vi "Read MAP data file.vi"(11 "Data folder":path) -> (2 "File name":string, 3 "Map data ref":refnum<data-value>, 4 "Error Out":errorcluster)   [LabVIEW 2022 SP3]
uses:
  Datatypes/Map graph data.ctl
  <vilib>/Utility/error.llb/Error Cluster From Error Code.vi
  <vilib>/ErrorRing/Error Ring.xnode
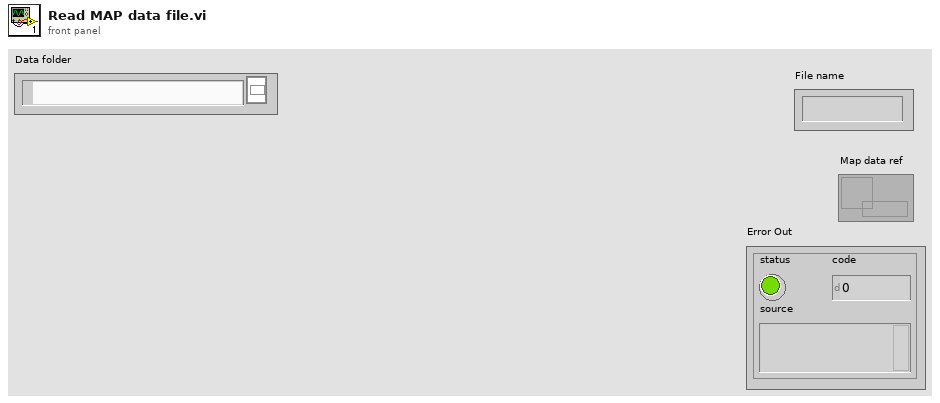
[diagram p1: front panel]
types:
  T1 = typedef "Map graph data.ctl" = cluster{"Field [T]":dbl[], "Intensity":dbl[][], "Start F [GHz]":dbl, "End F[GHz]":dbl, "BStart[T]":dbl, "Bend[T]":dbl, "Bsize":i32}
  T2 = enum16{"open", "open or create", "create or replace", "create", "open (read-only)"}
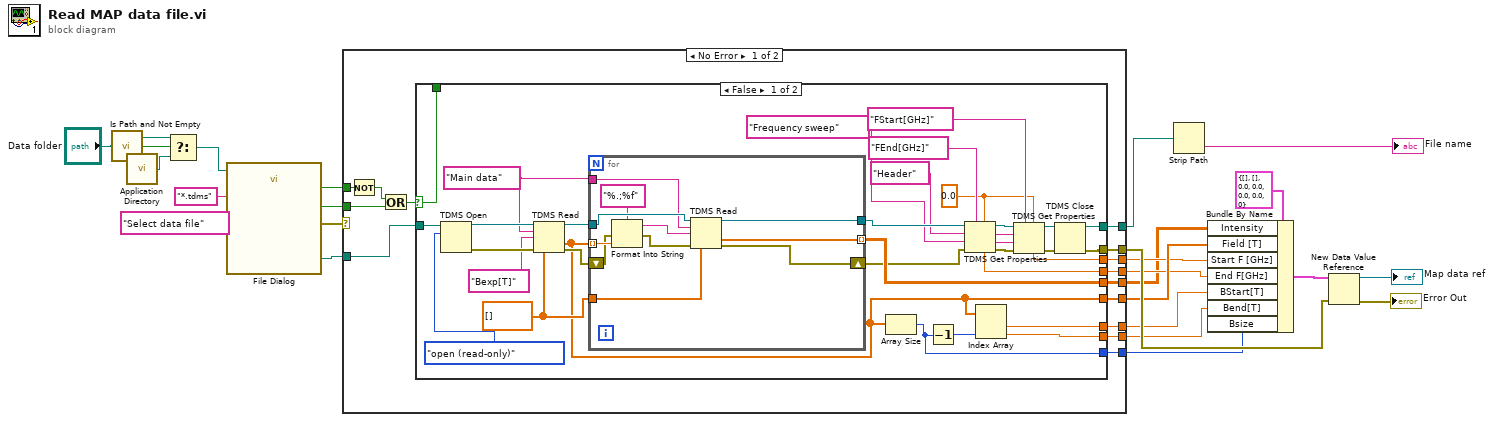
[diagram p0: block diagram]
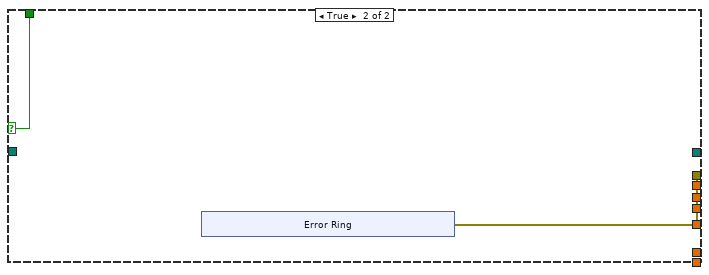
[diagram p2: hidden frame]
diagram:
  n1 = call <vilib>:"Is Path and Not Empty.vi"("path"="Data folder") -> ("Is Path and Not Empty?"=w18:bool)  [unwired: 4 in]
  n2 = call <vilib>:"Application Directory.vi"() -> ("Application Directory"=w15:path)
  n3 = Select(t="Data folder", s=w18, f=w15) -> (s? t:f=w16:path)
  n4 = call "File Dialog"("start path"=w16, "prompt"="Select data file", "pattern (all files)"="*.tdms") -> ("selected path"=w23:path, "exists"=w22:bool, "cancelled"=w21:bool, "error out"=w20:errorcluster)  [unwired: 9 in]
  n5 = case shown="No Error" w20 {
    selector: w20 -> [_ w89]
    tunnel: w23 -> [w38 _]
    tunnel: w22 -> [w37 _]
    tunnel: w21 -> [w34 _]
    tunnel: [w33 w89] -> w13
    tunnel: [w32 _] -> w11
    tunnel: [w31 _] -> w7
    tunnel: [w30 _] -> w9
    tunnel: [w29 _] -> w8
    tunnel: [w28 _] -> w6
    tunnel: [w27 _] -> w5
    tunnel: [w26 _] -> w4
    tunnel: [w25 _] -> w2
    frame No Error {
      n6 = Not(x=w37) -> (.not. x?=w36:bool)
      n7 = Or(x=w36, y=w34) -> (x .or. y?=w35:bool)
      n8 = case shown="False" w35 {
        selector: w35 -> [w71 w84]
        tunnel: w38 -> [w70 _]
        tunnel: [w71 w84] -> _
        tunnel: [w61 w83] -> w33
        tunnel: [w44 _] -> w32
        tunnel: [w60 _] -> w31
        tunnel: [w57 _] -> w29
        tunnel: [w46 _] -> w30
        tunnel: [w42 _] -> w28
        tunnel: [w41 _] -> w27
        tunnel: [w40 _] -> w26
        tunnel: [w39 _] -> w25
        frame False {
          w45 = "Main data"
          w47 = 0.0 ("Start F [GHz]")
          w64 = dbl[] []
          n9 = TDMS Open(10:T2."open (read-only)" ("operation (0:open)"), 11:w70) -> (0:w67:errorcluster, 3:w68:refnum<k34>)  [unwired: 5 in]
          n10 = TDMS Read(0:w68, 5:w45, 7:"Bexp[T]" ("channel name(s) in"), 11:w67, 12:w64) -> (4:w65:refnum<k34>, 10:w44:dbl[], 15:w63:errorcluster)  [unwired: 3 in, 3 out]
          n11 = for {
            tunnel: w65 -> [w79]
            tunnel: w44 -> [w82] mode=indexing
            tunnel: w64 -> [w74]
            tunnel: [w78] -> w60 mode=indexing
            tunnel: [w76] -> w62
            shift-right: [w77] -> w58
            shift-left: w63 -> [w75]
            tunnel: w45 -> [w73]
            n12 = Format Into String(format string="%.;%f", error in=w75, w82) -> (resulting string=w80:string, error out=w81:errorcluster)  [unwired: 1 in]
            n13 = TDMS Read(0:w79, 5:w73, 7:w80, 11:w81, 12:w74) -> (4:w76:refnum<k34>, 10:w78:dbl[], 15:w77:errorcluster)  [unwired: 3 in, 3 out]
          }
          n14 = Array Size(array=w44) -> (size(s)=w40:i32)
          n15 = Decrement(x=w40) -> (x-1=w43:i32)
          n16 = TDMS Get Properties(5:w47, 7:"FEnd[GHz]", 8:w58, 9:"Frequency sweep", 10:"Header" ("group name in"), 11:w62) -> (0:w52:errorcluster, 1:w48:string, 2:w49:string, 3:w59:refnum<k34>, 4:w57:dbl)  [unwired: 1 out]
          n17 = Index Array(array=w44, index #2=w43) -> (element #1=w42:dbl, element #2=w41:dbl)  [unwired: 1 in]
          n18 = TDMS Get Properties(5:w47, 7:"FStart[GHz]", 8:w52, 9:w48, 10:w49, 11:w59) -> (0:w53:errorcluster, 3:w54:refnum<k34>, 4:w46:dbl)  [unwired: 3 out]
          n19 = TDMS Close(8:w53, 11:w54) -> (0:w61:errorcluster, 3:w39:path)
        }
        frame True {
          n20 = xnode "Error Ring"() -> ("error out"=w83:errorcluster)
        }
      }
    }
    frame Error {
    }
  }
  n21 = Strip Path(path=w2) -> (name=→"File name":string)  [unwired: 1 out]
  n22 = Bundle By Name(cluster=T1 {"Field [T]"=[], "Intensity"=[], "Start F [GHz]"=0.0, "End F[GHz]"=0.0, "BStart[T]"=0.0, "Bend[T]"=0.0, "Bsize"=0} ("Cluster 2"), "Intensity"=w7, "Field [T]"=w11, "Start F [GHz]"=w9, "End F[GHz]"=w8, "BStart[T]"=w6, "Bend[T]"=w5, "Bsize"=w4) -> (w12:T1)
  n23 = New Data Value Reference(data value=w12, error in=w13) -> (data value reference=→"Map data ref":refnum<data-value>, error out=→"Error Out":errorcluster)
